vi "Get_PixelGapWidth.vi"(8 "error in":errorcluster, 11 "camera handle in":u64) -> (0 "error out":errorcluster, 1 "PixelGapWidth":dbl, 3 "camera handle out":u64)   [LabVIEW 2019, in "PICam.lvlib"]
doc: "Requests the time the sensor is exposed in milliseconds (mS)."
uses:
  PICam.lvlib
  Picam64.dll   
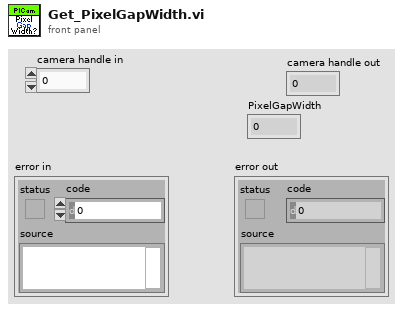
[diagram p1: front panel]
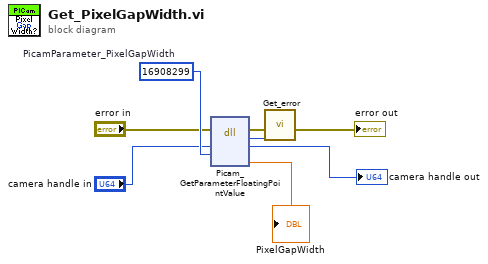
[diagram p0: block diagram]
diagram:
  w5 = u32 16908299  # PicamParameter_PixelGapWidth
  n1 = dll-call lib="Picam32.dll" fn="Picam_GetParameterFloatingPointValue"(error in="error in", "camera"="camera handle in", "PicamParameter"=w5) -> (error out=w8:errorcluster, "return type"=w1:i32, "camera"=→"camera handle out":u64, "PixelGapWidth"=→"PixelGapWidth":dbl)  [unwired: 4 in, 1 out]
  n2 = call "Get_error.vi"("PICam_Error"=w1, "error in (no error)"=w8) -> ("error out"=→"error out":errorcluster)  [unwired: 9 in]
